vi "From Variant.vi"(8 "Error In":errorcluster, 10 "Variant":variant, 11 "TD Int In":refnum<class "Int.lvclass">) -> (0 "Error Out":errorcluster, 3 "TD Int Out":refnum<class "Int.lvclass">)   [LabVIEW 2017, in "Tree API.lvlib" / "Int.lvclass"]
doc: "Dynamic dispatch interface for conversion of variant LV data to Tree Data classes."
uses:
  Int.lvclass
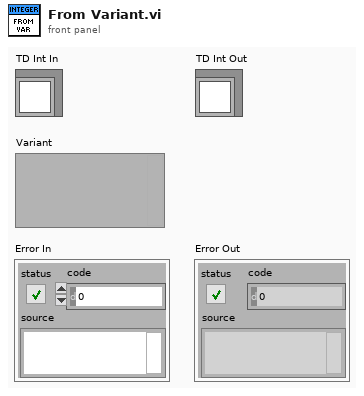
[diagram p1: front panel]
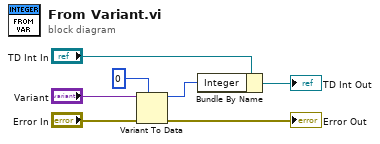
[diagram p0: block diagram]
diagram:
  n1 = Variant To Data(error in="Error In", type=i64 0 ("Integer"), Variant="Variant") -> (data=w2:i64, error out=→"Error Out":errorcluster)
  n2 = Bundle By Name(cluster="TD Int In", "Integer"=w2) -> (→"TD Int Out":refnum<class "Int.lvclass">)
